vi "BeamProfiler.vi"() -> ()   [LabVIEW 2014]
uses:
  <vilib>/Analysis/6fits.llb/Curve Fitting Criteria.ctl
  <vilib>/vision/Image Controls.llb/IMAQ Rounding Mode.ctl
  <vilib>/vision/Image Controls.llb/IMAQ Image.ctl
  <vilib>/vision/NI_Vision_Development_Module.lvlib
  <vilib>/ptbypt/NI_PtbyPt.lvlib
  <vilib>/Analysis/NI_AALPro.lvlib
panel:
  in  "resample":dbl=1.0
  in  "Smooth":bool
  in  "max proj":bool
  in  "average":dbl=1.0
  in  "centroid":bool
  out "Temp":dbl format="%#_2g"
  out "fps":dbl
  in  "Exposure Time (ms)":dbl(slide)=32000.0 caption="Exposure Time" min=2000.0 max=32000.0 scale=2000.0..32000.0 scale format="%^#_3g"
  in  "Gain":dbl(slide)=1.0 min=1.0 max=4.0 scale=1.0..4.0
  in  "Auto":bool
  in  "Contrast":i64(slide) caption="Gain (Raw)" min=0 max=384 step=1 scale=0.0..100.0
  in  "Gamma":dbl(slide)=0.5 min=0.5 max=2.0 step=0.1 scale=0.5..2.0
  in  "Auto":bool
  out "Beam profile":T1(plugin-control)
  in  "zero":bool
  in  "mmPerPx":dbl=0.0059
  out "XY Center location":cluster{"Array":dbl[], "Array 3":dbl[]}(graph)
  out "Y center (px)":dbl
  out "X center (px)":dbl
  in  "Center\n Color":u32(colorbox)=10735
  in  "Black\n zero":bool=TRUE
  in  "Operator":T2(ring)=enum."Clear  if < "
  out "X Histogram":cluster{"X":dbl, "Y":dbl}[](graph)
  out "Y Histogram":cluster{"X":dbl, "Y":dbl}[](graph)
  in  "Palette Number (gray)":T3(ring)=enum."Rainbow"
  in  "Decrease":bool
  in  "Increase":bool
  in  "zoom 4":bool
  in  "zoom 3":bool
  in  "zoom 2":bool
  in  "zoom1":bool
  in  "stop":bool
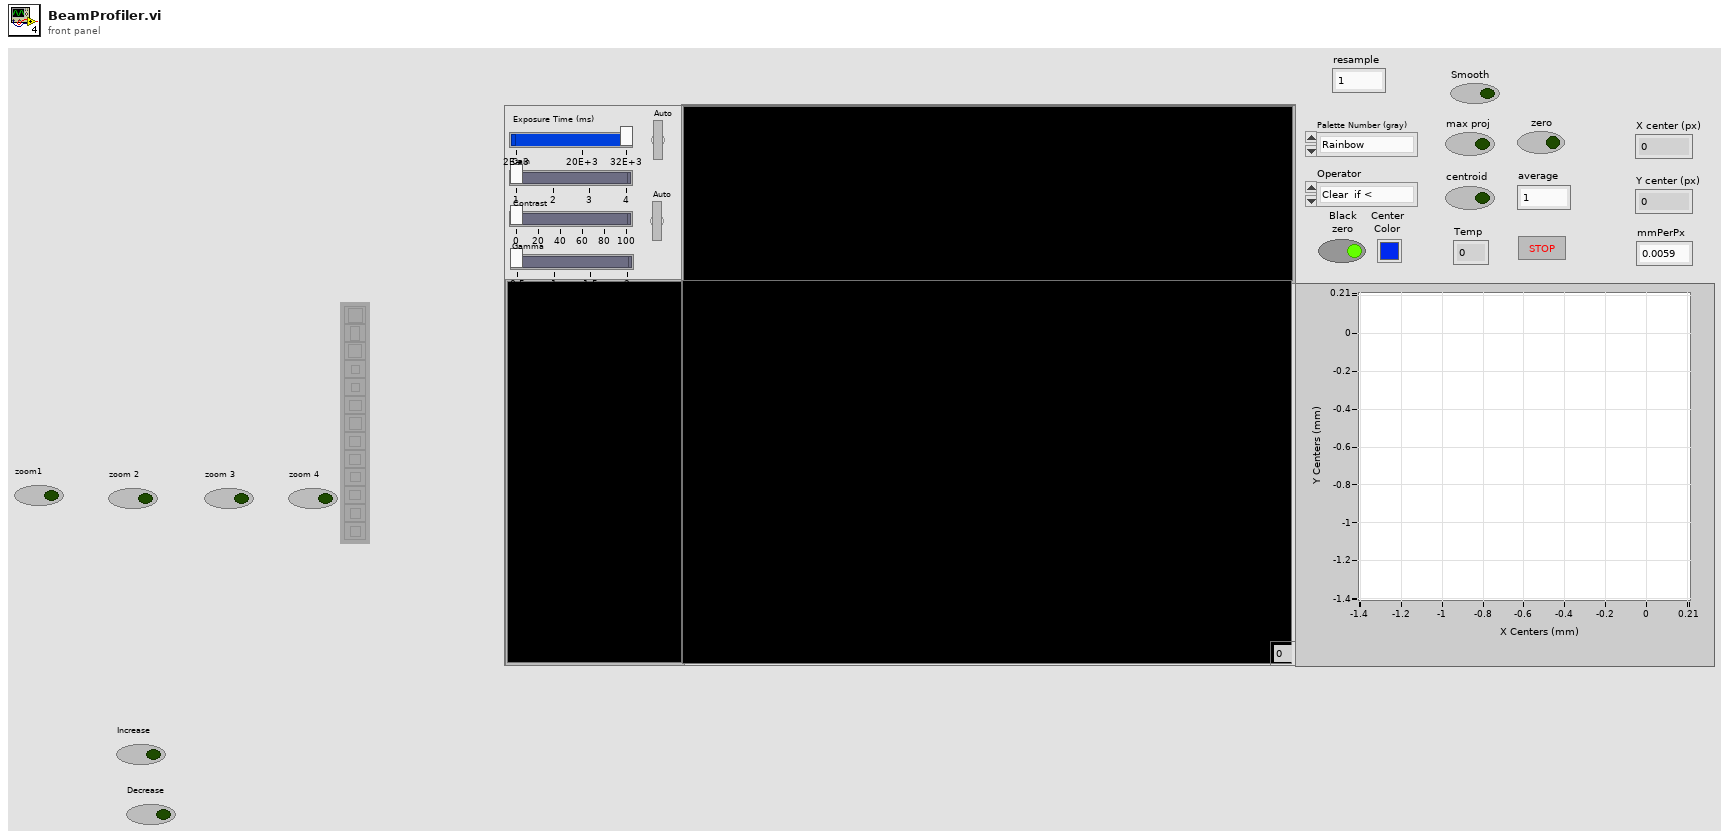
[diagram p1: front panel]
types:
  T1 = typedef "IMAQ Image.ctl" = refnum<image>
  T2 = enum32{"Average", "Min", "Max", "Clear  if < ", "Clear  if < or =", "Clear  if =", "Clear  if > or =", "Clear  if >"}
  T3 = enum32{"Gray", "Binary", "Gradient", "Rainbow", "Temperature"}
  T4 = typedef "Image Type" = u32
  T5 = typedef "IMAQ Rounding Mode.ctl" = enum16{"Optimize", "Truncate"}
  T6 = cluster{"Brightness":sgl, "Contrast":sgl, "Gamma":sgl}
  T7 = typedef "NI_AALPro.lvlib/Curve Fitting Criteria.ctl" = u16
  T8 = typedef "LVRangeTypeDef.ctl" = cluster{"Minimum":dbl, "Maximum":dbl, "Increment":dbl, "Minor Increment":dbl, "Start":dbl}
  T9 = cluster{"Mean Value":sgl, "Standard Variation":sgl, "Minimal Value":sgl, "Maximal Value":sgl, "Area (calibrated)":sgl, "Area (pixels)":u32, "%":sgl, "Calibration Valid":bool}
  T10 = typedef "ROI Descriptor" = cluster{"Global Rectangle":i32[], "Contours":cluster{"ID":enum32{"External", "Internal"}, "Type":u32, "Coordinates":i32[]}[]}
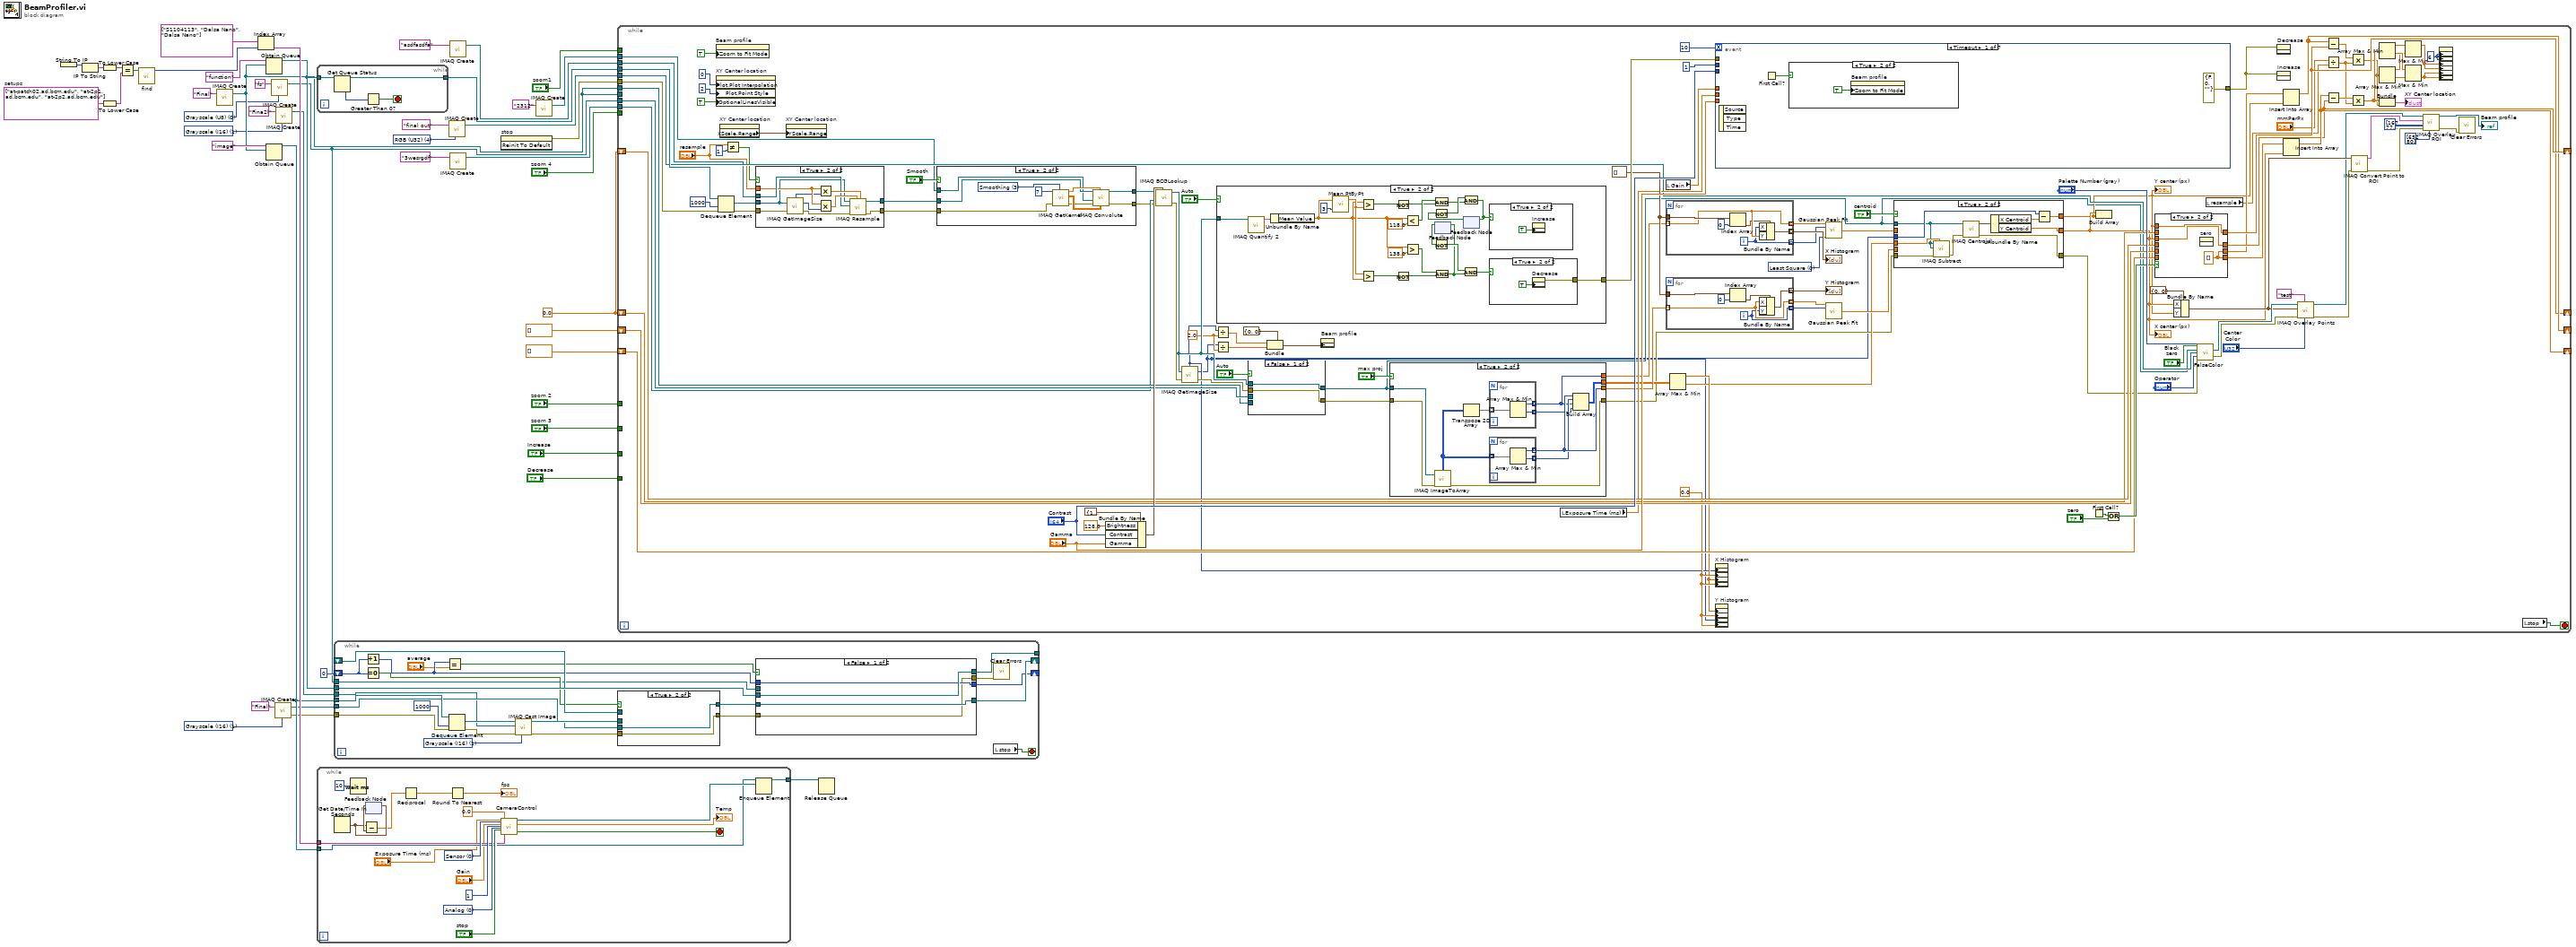
[diagram p0: block diagram]
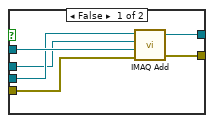
[diagram p2: hidden frame]
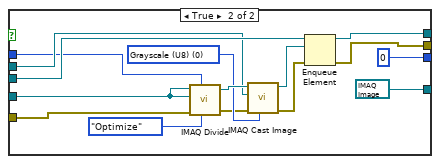
[diagram p3: hidden frame]
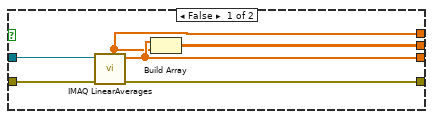
[diagram p6: hidden frame]
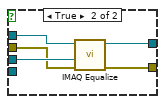
[diagram p9: hidden frame]
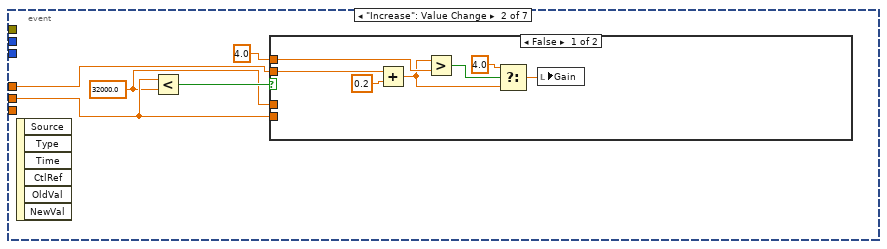
[diagram p14: hidden frame]
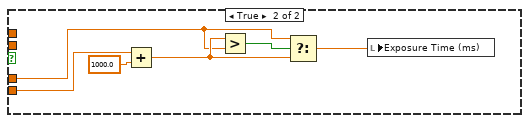
[diagram p15: hidden frame]
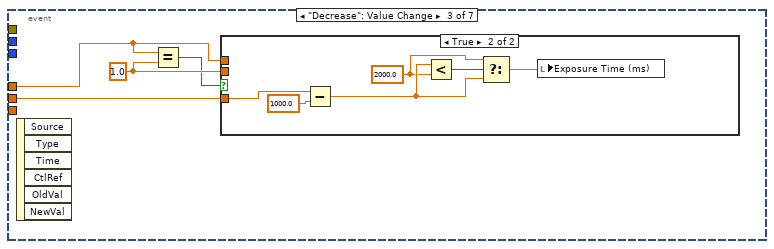
[diagram p16: hidden frame]
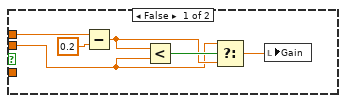
[diagram p17: hidden frame]
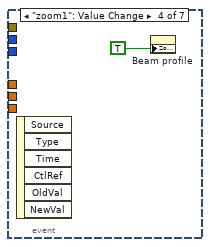
[diagram p18: hidden frame]
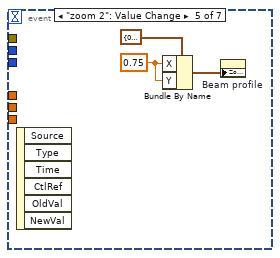
[diagram p19: hidden frame]
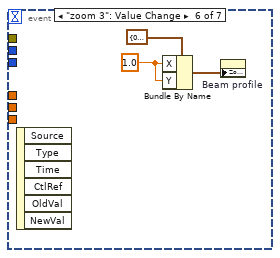
[diagram p20: hidden frame]
diagram:
  w9 = T4 0 items=["Grayscale (U8)", "Grayscale (I16)", "Grayscale (SGL)", "Complex (CSG)", "RGB (U32)", "HSL (U32)", "RGB (U64)", "Grayscale (U16)"] ("Image Type")
  w14 = T4 1 items=["Grayscale (U8)", "Grayscale (I16)", "Grayscale (SGL)", "Complex (CSG)", "RGB (U32)", "HSL (U32)", "RGB (U64)", "Grayscale (U16)"] ("Image Type")
  w16 = T4 1 items=["Grayscale (U8)", "Grayscale (I16)", "Grayscale (SGL)", "Complex (CSG)", "RGB (U32)", "HSL (U32)", "RGB (U64)", "Grayscale (U16)"] ("Image Type")
  w25 = T4 4 items=["Grayscale (U8)", "Grayscale (I16)", "Grayscale (SGL)", "Complex (CSG)", "RGB (U32)", "HSL (U32)", "RGB (U64)", "Grayscale (U16)"] ("Image Type")
  w29 = 0.0
  w36 = string[] ["at-patch02.ad.bcm.edu", "at-2p1.ad.bcm.edu", "at-2p2.ad.bcm.edu"]  # setups
  n1 = String To IP() -> (0:w39:u32)  [unwired: 1 in]
  n2 = IP To String(2:w39) -> (0:w38:string)  [unwired: 1 in]
  n3 = To Lower Case(string=w38) -> (all lower case string=w37:string)
  n4 = To Lower Case(string=w36) -> (all lower case string=w35:string[])
  n5 = Equal?(x=w37, y=w35) -> (x = y?=w34:bool[])
  n6 = call "find.vi"("Array"=w34) -> ("Index"=w33:i32)  [unwired: 10 in]
  n7 = call "IMAQ Create"("Image Name"="Final") -> ("New Image"=w18:T1)  [unwired: 4 in, 1 out]
  n8 = Index Array(array=string[] ["S1104113", "Dalsa Nano", "Dalsa Nano"], index=w33) -> (element=w28:string)
  n9 = Obtain Queue(name (unnamed)="function", element data type=w18) -> (queue out=w19:refnum<queue>)  [unwired: 3 in, 2 out]
  n10 = Obtain Queue(name (unnamed)="image", element data type=w18) -> (queue out=w20:refnum<queue>)  [unwired: 3 in, 2 out]
  n11 = call "IMAQ Create"("Image Name"="fs", "Image Type"=w9) -> ("New Image"=w8:T1)  [unwired: 3 in, 1 out]
  n12 = call "IMAQ Create"("Image Name"="Final", "Image Type"=w16) -> ("New Image"=w15:T1, "error out"=w7:errorcluster)  [unwired: 3 in]
  n13 = call "IMAQ Create"("Image Name"="Fina2l", "Image Type"=w14) -> ("New Image"=w12:T1)  [unwired: 3 in, 1 out]
  n14 = while {
    tunnel: w19 -> [w51]
    tunnel: [w50] -> w22
    stop <- w49 stop-if-true
    n15 = Get Queue Status(queue=w51) -> (queue out=w50:refnum<queue>, # elements in queue=w48:i32)  [unwired: 2 in, 6 out]
    n16 = Greater Than 0?(x=w48) -> (x > 0?=w49:bool)
  }
  n17 = while {
    tunnel: w28 -> [w65]
    tunnel: w20 -> [w62]
    tunnel: [w61] -> w27
    stop <- w64 stop-if-true
    w67 = u32 0 items=["Analog"] ("Black Level Selector")
    w66 = u32 0 items=["Sensor", "Digital"] ("Gain Selector")
    n18 = Get Date/Time In Seconds() -> (seconds since 1Jan1904=w56:timestamp)
    n19 = Wait (ms)(milliseconds to wait=u32 10) -> ()  [unwired: 1 out]
    n20 = feedback #1() -> (w57:timestamp)  [unwired: 1 in]
    n21 = Subtract(x=w56, y=w57) -> (x-y=w55:dbl)
    n22 = feedback-in #1(w56) -> ()
    n23 = Reciprocal(x=w55) -> (1/x=w58:dbl)
    n24 = Round To Nearest(number=w58) -> (nearest integer value=→"fps":dbl)
    n25 = call "CameraControl.vi"("Exposure Time"="Exposure Time (ms)", "Gain Selector"=w66, "Gain"="Gain", "Gain (Raw)"=i64 1, "Black Level Selector"=w67, "Stop (F)"="stop", "Black Level"=0.0, "Camera"=w65) -> ("Image Out"=w63:T1, "Temp"=→"Temp":dbl, "Stopped"=w64:bool)  [unwired: 14 in, 3 out]
    n26 = Enqueue Element(queue=w62, element=w63) -> (queue out=w61:refnum<queue>)  [unwired: 2 in, 2 out]
  }
  n27 = while {
    tunnel: w19 -> [w93]
    tunnel: w20 -> [w94]
    tunnel: [w92] -> _
    shift-right: [w84] -> _
    shift-left: _ -> [w91]
    tunnel: w15 -> [w90]
    tunnel: w12 -> [w87]
    shift-right: [w83] -> _
    shift-left: 0 -> [w79]
    tunnel: w8 -> [w77]
    tunnel: w7 -> [w75]
    stop <- w95 stop-if-true
    w86 = T4 1 items=["Grayscale (U8)", "Grayscale (I16)", "Grayscale (SGL)", "Complex (CSG)", "RGB (U32)", "HSL (U32)", "RGB (U64)", "Grayscale (U16)"] ("Image Type")
    n28 = Increment(x=w79) -> (x+1=w80:i32)
    n29 = Equal To 0?(x=w79) -> (x = 0?=w82:bool)
    n30 = Equal?(x=w80, y="average") -> (x = y?=w81:bool)
    n31 = Dequeue Element(queue=w94, timeout in ms (-1)=1000, error in (no error)=w75) -> (element=w88:T1, error out=w74:errorcluster)  [unwired: 2 out]
    n32 = call "IMAQ Cast Image"("Image Type"=w86, "error in (no error)"=w74, "Image Dst"=w87, "Image Src"=w88) -> ("error out"=w73:errorcluster, "Image Dst Out"=w89:T1)  [unwired: 6 in]
    n33 = case shown="True" w82 {
      tunnel: w89 -> [w100 w103]
      tunnel: [w99 w103] -> w85
      tunnel: w91 -> [w101 _]
      tunnel: w90 -> [w98 _]
      tunnel: w73 -> [w97 w102]
      tunnel: [w96 w102] -> w72
      frame False {
        n34 = call "IMAQ Add"("Image Src A"=w100, "Image Dst"=w98, "Image Src B"=w101, "error in (no error)"=w97) -> ("Image Dst Out"=w99:T1, "error out"=w96:errorcluster)  [unwired: 3 in]
      }
      frame True {
      }
    }
    n35 = case shown="False" w81 {
      tunnel: w93 -> [w107 w122]
      tunnel: [w107 w121] -> w92
      tunnel: w85 -> [w106 w112]
      tunnel: [w106 T1 refnum ("Image Dst Out")] -> w84
      tunnel: w80 -> [w105 w113]
      tunnel: [w105 0] -> w83
      tunnel: w77 -> [_ w114]
      tunnel: w72 -> [w104 w111]
      tunnel: [w104 w108] -> w71
      frame False {
      }
      frame True {
        w115 = T4 0 items=["Grayscale (U8)", "Grayscale (I16)", "Grayscale (SGL)", "Complex (CSG)", "RGB (U32)", "HSL (U32)", "RGB (U64)", "Grayscale (U16)"] ("Image Type")
        n36 = call "IMAQ Divide"("Image Src A"=w112, "Constant"=w113, "Image Dst"=w112, "Rounding Mode"=IMAQ_Rounding_Mode."Optimize", "error in (no error)"=w111) -> ("Image Dst Out"=w116:T1, "error out"=w110:errorcluster)  [unwired: 2 in]
        n37 = call "IMAQ Cast Image"("Image Type"=w115, "error in (no error)"=w110, "Image Dst"=w114, "Image Src"=w116) -> ("error out"=w109:errorcluster, "Image Dst Out"=w117:T1)  [unwired: 6 in]
        n38 = Enqueue Element(queue=w122, element=w117, error in (no error)=w109) -> (queue out=w121:refnum<queue>, error out=w108:errorcluster)  [unwired: 1 in, 1 out]
      }
    }
    n39 = call <vilib>:"Clear Errors.vi"("error in (no error)"=w71) -> ()  [unwired: 5 in, 2 out]
    n40 = local read "stop"() -> (w95:bool)
  }
  n41 = call "IMAQ Create"("Image Name"="final out", "Image Type"=w25) -> ("New Image"=w23:T1)  [unwired: 3 in, 1 out]
  n42 = call "IMAQ Create"("Image Name"="asdfasdfa") -> ("New Image"=w1:T1)  [unwired: 4 in, 1 out]
  n43 = call "IMAQ Create"("Image Name"="3wesrgdf") -> ("New Image"=w5:T1)  [unwired: 4 in, 1 out]
  n44 = invoke on="stop" class="Bool (strict)" method="Reinit To Default"() -> (error out=w40:errorcluster)  [unwired: 3 in, 2 out]
  n45 = call "IMAQ Create"("Image Name"="2312") -> ("New Image"=w3:T1)  [unwired: 4 in, 1 out]
  n46 = while {
    tunnel: "zoom1" -> [_]
    tunnel: "zoom 4" -> [_]
    tunnel: "zoom 2" -> [_]
    tunnel: "zoom 3" -> [_]
    tunnel: "Increase" -> [_]
    tunnel: "Decrease" -> [_]
    tunnel: w18 -> [w146]
    tunnel: w40 -> [w149]
    shift-right: [w201] -> _
    shift-left: dbl[] [] -> [w190]
    shift-right: [w199] -> _
    shift-left: dbl[] [] -> [w192]
    shift-right: [w198] -> _
    shift-left: w29 -> [w202]
    shift-right: [w200] -> _
    shift-left: w29 -> [w203]
    tunnel: w22 -> [w175]
    tunnel: w23 -> [w174]
    tunnel: w18 -> [_]
    tunnel: w8 -> [w164]
    tunnel: w5 -> [w145]
    tunnel: w3 -> [w141]
    tunnel: w1 -> [w136]
    stop <- w176 stop-if-true
    w127 = 2.0 ("y")
    w172 = 0.0 ("X Scale.Range:Minimum")
    w188 = u8 6 ("X Scale.Mapping Mode")
    w193 = T7 0 items=["Least Square", "Least Absolute Residual", "Bisquare"] ("method")
    w226 = cluster{"X":dbl, "Y":dbl}[] [] ("XY Graph")
    n47 = property on="Beam profile" class="ImageControl"("Zoom to Fit Mode"=TRUE) -> ()  [unwired: 2 in, 2 out]
    n48 = property on="XY Center location" class="XYGraph (strict)"("Plot.Plot Interpolation"=u8 0, "Plot.Point Style"=u8 2 ("Cursor.Cursor Point Style"), "OptionalLinesVisible"=TRUE ("Cartesian Lines:Visible")) -> ()  [unwired: 2 in, 2 out]
    n49 = Dequeue Element(queue=w175, timeout in ms (-1)=1000, error in (no error)=w149) -> (element=w138:T1, error out=w131:errorcluster)  [unwired: 2 out]
    n50 = property on="XY Center location" class="XYGraph (strict)"() -> ("XScale.Range"=w173:T8)  [unwired: 2 in, 2 out]
    n51 = Not Equal?(x="resample", y=1) -> (x != y?=w133:bool)
    n52 = case shown="True" w133 {
      tunnel: w138 -> [w241 w244]
      tunnel: [w241 w252] -> w140
      tunnel: w131 -> [w240 w243]
      tunnel: [w240 w251] -> w139
      tunnel: w136 -> [_ w248]
      tunnel: "resample" -> [_ w247]
      frame False {
      }
      frame True {
        n53 = call "IMAQ GetImageSize"("Image"=w244, "error in (no error)"=w243) -> ("Y Resolution"=w245:i32, "X Resolution"=w246:i32, "error out"=w242:errorcluster)  [unwired: 2 in]
        n54 = Multiply(x=w247, y=w246) -> (x*y=w249:dbl)
        n55 = Multiply(x=w247, y=w245) -> (x*y=w250:dbl)
        n56 = call "IMAQ Resample"("X Resolution"=w249, "Y Resolution"=w250, "error in (no error)"=w242, "Image Dst"=w248, "Image Src"=w244) -> ("error out"=w251:errorcluster, "Image Dst Out"=w252:T1)  [unwired: 5 in]
      }
    }
    n57 = property on="XY Center location" class="XYGraph (strict)"("YScale.Range"=w173) -> ()  [unwired: 2 in, 2 out]
    n58 = case shown="True" "Smooth" {
      tunnel: [w254 w261] -> w144
      tunnel: w139 -> [w254 w260]
      tunnel: [w253 w258] -> w143
      tunnel: w140 -> [w253 w259]
      tunnel: w141 -> [_ w256]
      frame False {
      }
      frame True {
        w255 = u16 3 items=["Gradient"=1, "Laplacian"=2, "Smoothing"=3, "Gaussian"=4] ("Kernel Family")
        n59 = call "IMAQ GetKernel"("Kernel Family"=w255, "error in (no error)"=w260, "Kernel Size (3,5,...)"=7) -> ("error out"=w262:errorcluster, "Kernel"=w264:sgl[][], "Divider"=w263:sgl)  [unwired: 5 in, 1 out]
        n60 = call "IMAQ Convolute"("Kernel"=w264, "Divider (kernel sum)"=w263, "error in (no error)"=w262, "Image Dst"=w256, "Image Src"=w259) -> ("error out"=w261:errorcluster, "Image Dst Out"=w258:T1)  [unwired: 5 in]
      }
    }
    n61 = Bundle By Name(cluster=T6 {"Brightness"=128.0, "Contrast"=45.0, "Gamma"=1.0} ("BCG Values"), "Brightness"=sgl 128.0, "Contrast"="Contrast", "Gamma"="Gamma") -> (w230:T6)
    n62 = call "IMAQ BCGLookup"("Image Src"=w143, "BCG Values"=w230, "Image Dst"=w145, "error in (no error)"=w144) -> ("Image Dst Out"=w147:T1, "error out"=w148:errorcluster)  [unwired: 3 in]
    n63 = call "IMAQ GetImageSize"("Image"=w147, "error in (no error)"=w148) -> ("Y Resolution"=w123:i32, "X Resolution"=w124:i32, "error out"=w157:errorcluster)  [unwired: 2 in]
    n64 = Divide(x=w124, y=w127) -> (x/y=w126:dbl)
    n65 = Divide(x=w123, y=w127) -> (x/y=w125:dbl)
    n66 = case shown="True" "Auto" {
      tunnel: w147 -> [_ w347]
      tunnel: [_ w345] -> w237
      frame False {
      }
      frame True {
        n67 = call "IMAQ Quantify 2"("Image"=w347) -> ("Global Report"=w343:T9)  [unwired: 8 in, 2 out]
        n68 = Unbundle By Name(w343) -> ("Mean Value"=w335:sgl)
        n69 = call <vilib>:"Mean PtByPt.vi"("x"=w335, "sample length"=3) -> ("mean"=w336:dbl)  [unwired: 2 in, 1 out]
        n70 = Greater?(x=w335, y=w336) -> (0:w340:bool)
        n71 = Greater?(x=w336, y=w335) -> (0:w337:bool)
        n72 = Not(x=w340) -> (.not. x?=w339:bool)
        n73 = Not(x=w337) -> (.not. x?=w338:bool)
        n74 = Less?(x=w335, y=sgl 118.0) -> (x < y?=w342:bool)
        n75 = Greater?(x=w335, y=sgl 138.0) -> (0:w328:bool)
        n76 = And(x=w342, y=w339) -> (x .and. y?=w332:bool)
        n77 = feedback #2() -> (w329:bool)  [unwired: 1 in]
        n78 = Not(x=w329) -> (.not. x?=w330:bool)
        n79 = And(x=w328, y=w338) -> (x .and. y?=w327:bool)
        n80 = feedback-in #2(w327) -> ()
        n81 = And(x=w330, y=w327) -> (x .and. y?=w326:bool)
        n82 = feedback #3() -> (w334:bool)  [unwired: 1 in]
        n83 = Not(x=w334) -> (.not. x?=w333:bool)
        n84 = And(x=w333, y=w332) -> (x .and. y?=w331:bool)
        n85 = feedback-in #3(w331) -> ()
        n86 = case shown="True" w331 {
          frame False {
          }
          frame True {
            n87 = property on="Increase" class="Bool (strict)"("Val(Sgnl)"=TRUE ("Value (Signaling)")) -> ()  [unwired: 2 in, 2 out]
          }
        }
        n88 = case shown="True" w326 {
          tunnel: [_ w349] -> w345
          frame False {
          }
          frame True {
            n89 = property on="Decrease" class="Bool (strict)"("Val(Sgnl)"=TRUE ("Value (Signaling)")) -> (error out=w349:errorcluster)  [unwired: 2 in, 1 out]
          }
        }
      }
    }
    n90 = case shown="False" "Auto" {
      tunnel: [w320 w324] -> w159
      tunnel: w147 -> [w320 w325]
      tunnel: w146 -> [_ _]
      tunnel: w164 -> [_ w323]
      tunnel: w157 -> [w319 w322]
      tunnel: [w319 w321] -> w156
      frame False {
      }
      frame True {
        n91 = call "IMAQ Equalize"("error in (no error)"=w322, "Image Dst"=w323, "Image Src"=w325) -> ("error out"=w321:errorcluster, "Image Dst Out"=w324:T1)  [unwired: 7 in]
      }
    }
    n92 = Bundle(cluster=cluster{"X":u32, "Y":u32} {"X"=0, "Y"=0} ("Image Center Position:All Elements"), "X"=w126, "Y"=w125) -> (w128:cluster{"X":u32, "Y":u32})
    n93 = property on="Beam profile" class="ImageControl"("Image Center Position"=w128) -> ()  [unwired: 2 in, 2 out]
    n94 = case shown="True" "max proj" {
      tunnel: [w268 w275] -> w162
      tunnel: [w269 w277] -> w161
      tunnel: w159 -> [w270 w280]
      tunnel: [w267 w273] -> w158
      tunnel: w156 -> [w266 w272]
      tunnel: [w265 w271] -> w155
      frame False {
        n95 = call "IMAQ LinearAverages"("error in (no error)"=w266, "Image Src"=w270) -> ("error out"=w265:errorcluster, "Y Axis Averages"=w269:sgl[], "X Axis Averages"=w268:sgl[])  [unwired: 5 in, 2 out]
        n96 = Build Array(w269, w268) -> (w267:sgl[][])
      }
      frame True {
        n97 = call "IMAQ ImageToArray"("error in (no error)"=w272, "Image"=w280) -> ("error out"=w271:errorcluster, "Image Pixels (U8)"=w279:u8[][])  [unwired: 2 in, 3 out]
        n98 = Transpose 2D Array(2D array=w279) -> (transposed array=w278:u8[][])
        n99 = for {
          tunnel: w278 -> [w283] mode=indexing
          tunnel: [w282] -> w275 mode=indexing
          tunnel: [w281] -> w274 mode=indexing
          n100 = Array Max & Min(array=w283) -> (max value=w282:u8, min value=w281:u8)  [unwired: 2 out]
        }
        n101 = for {
          tunnel: w279 -> [w286] mode=indexing
          tunnel: [w285] -> w277 mode=indexing
          tunnel: [w284] -> w276 mode=indexing
          n102 = Array Max & Min(array=w286) -> (max value=w285:u8, min value=w284:u8)  [unwired: 2 out]
        }
        n103 = Build Array(w277, w276, w275, w274) -> (w273:u8[][])
      }
    }
    n104 = local read "Exposure Time (ms)"() -> (w179:dbl)
    n105 = local read "Gain"() -> (w178:dbl)
    n106 = for {
      tunnel: w226 -> [w312]
      tunnel: w162 -> [w309] mode=indexing
      tunnel: [w310] -> w227 mode=indexing
      tunnel: [w309] -> w214 mode=indexing
      tunnel: [w308] -> w213 mode=indexing
      i -> [w308]
      n107 = Index Array(array=w312, index=0) -> (element=w307:cluster{"X":dbl, "Y":dbl})
      n108 = Bundle By Name(cluster=w307, "X"=w308, "Y"=w309) -> (w310:cluster{"X":dbl, "Y":dbl})
    }
    "X Histogram" <- w227
    n109 = for {
      tunnel: w226 -> [w318]
      tunnel: w161 -> [w314] mode=indexing
      tunnel: [w315] -> w228 mode=indexing
      tunnel: [w314] -> w212 mode=indexing
      tunnel: [w313] -> w211 mode=indexing
      i -> [w313]
      n110 = Index Array(array=w318, index=0) -> (element=w316:cluster{"X":dbl, "Y":dbl})
      n111 = Bundle By Name(cluster=w316, "X"=w314, "Y"=w313) -> (w315:cluster{"X":dbl, "Y":dbl})
    }
    "Y Histogram" <- w228
    n112 = Array Max & Min(array=w158) -> (max value=w166:sgl, min value=w163:sgl)  [unwired: 2 out]
    n113 = event shown="[0] Timeout" {
      selector: _ -> [_ _ _ _ _ _ _]
      dyn-events: _ -> [_ _ _ _ _ _ _]
      timeout: 10 -> [_ _ _ _ _ _ _]
      tunnel: w179 -> [_ w356 w373 _ _ _ _]
      tunnel: i64 1 ("Gain (Raw)") -> [_ _ _ _ _ _ _]
      tunnel: w178 -> [_ w358 w374 _ _ _ _]
      tunnel: "Contrast" -> [_ _ _ _ _ _ _]
      tunnel: "Gamma" -> [_ _ _ _ _ _ _]
      tunnel: [errorcluster {"status"=FALSE, "code"=0, "source"=""} ("error out") _ _ _ _ _ _] -> w238
      tunnel: w237 -> [_ _ _ _ _ _ _]
      event Timeout {
        n114 = event-data() -> ()  [unwired: 1 in, 3 out]
        n115 = First Call?() -> (First Call?: T/F=w351:bool)
        n116 = case shown="True" w351 {
          frame False {
          }
          frame True {
            n117 = property on="Beam profile" class="ImageControl"("Zoom to Fit Mode"=TRUE) -> ()  [unwired: 2 in, 2 out]
          }
        }
      }
      event "Increase": Value Change {
        w354 = 32000.0 ("y")
        n118 = event-data() -> ()  [unwired: 1 in, 6 out]
        n119 = Less?(x=w356, y=w354) -> (x < y?=w355:bool)
        n120 = case shown="False" w355 {
          tunnel: w356 -> [_ w371]
          tunnel: w358 -> [w365 _]
          tunnel: 4.0 ("y") -> [w363 _]
          tunnel: w354 -> [_ w366]
          frame False {
            n121 = Add(x=w365, y=0.2) -> (x+y=w361:dbl)
            n122 = Greater?(x=w361, y=w363) -> (0:w362:bool)
            n123 = Select(t=4.0, s=w362, f=w361) -> (s? t:f=w359:dbl)
            n124 = local write "Gain"(w359) -> ()
          }
          frame True {
            n125 = Add(x=w371, y=1000.0) -> (x+y=w368:dbl)
            n126 = Greater?(x=w368, y=w366) -> (0:w369:bool)
            n127 = Select(t=w366, s=w369, f=w368) -> (s? t:f=w367:dbl)
            n128 = local write "Exposure Time (ms)"(w367) -> ()
          }
        }
      }
      event "Decrease": Value Change {
        w375 = 1.0 ("y")
        n129 = event-data() -> ()  [unwired: 1 in, 6 out]
        n130 = Equal?(x=w374, y=w375) -> (x = y?=w372:bool)
        n131 = case shown="True" w372 {
          tunnel: w373 -> [_ w387]
          tunnel: w374 -> [w381 _]
          tunnel: w375 -> [w376 _]
          frame False {
            n132 = Subtract(x=w381, y=0.2) -> (x-y=w378:dbl)
            n133 = Less?(x=w378, y=w376) -> (x < y?=w379:bool)
            n134 = Select(t=w376, s=w379, f=w378) -> (s? t:f=w377:dbl)
            n135 = local write "Gain"(w377) -> ()
          }
          frame True {
            w383 = 2000.0 ("y")
            n136 = Subtract(x=w387, y=1000.0) -> (x-y=w384:dbl)
            n137 = Less?(x=w384, y=w383) -> (x < y?=w385:bool)
            n138 = Select(t=w383, s=w385, f=w384) -> (s? t:f=w382:dbl)
            n139 = local write "Exposure Time (ms)"(w382) -> ()
          }
        }
      }
      event "zoom1": Value Change {
        n140 = event-data() -> ()  [unwired: 1 in, 6 out]
        n141 = property on="Beam profile" class="ImageControl"("Zoom to Fit Mode"=TRUE) -> ()  [unwired: 2 in, 2 out]
      }
      event "zoom 2": Value Change {
        w389 = 0.75
        n142 = event-data() -> ()  [unwired: 1 in, 6 out]
        n143 = Bundle By Name(cluster=cluster{"X":sgl, "Y":sgl} {"X"=0.0, "Y"=0.0} ("ZoomSingle:All Elements"), "X"=w389, "Y"=w389) -> (w391:cluster{"X":sgl, "Y":sgl})
        n144 = property on="Beam profile" class="ImageControl"("ZoomSingle"=w391) -> ()  [unwired: 2 in, 2 out]
      }
      event "zoom 3": Value Change {
        w392 = 1.0
        n145 = event-data() -> ()  [unwired: 1 in, 6 out]
        n146 = Bundle By Name(cluster=cluster{"X":sgl, "Y":sgl} {"X"=0.0, "Y"=0.0} ("ZoomSingle:All Elements"), "X"=w392, "Y"=w392) -> (w394:cluster{"X":sgl, "Y":sgl})
        n147 = property on="Beam profile" class="ImageControl"("ZoomSingle"=w394) -> ()  [unwired: 2 in, 2 out]
      }
      event "zoom 4": Value Change {
        w395 = 1.5
        n148 = event-data() -> ()  [unwired: 1 in, 6 out]
        n149 = Bundle By Name(cluster=cluster{"X":sgl, "Y":sgl} {"X"=0.0, "Y"=0.0} ("ZoomSingle:All Elements"), "X"=w395, "Y"=w395) -> (w397:cluster{"X":sgl, "Y":sgl})
        n150 = property on="Beam profile" class="ImageControl"("ZoomSingle"=w397) -> ()  [unwired: 2 in, 2 out]
      }
    }
    n151 = property on="X Histogram" class="XYGraph (strict)"("XScale.Maximum"=w124, "XScale.Minimum"=w172, "YScale.Maximum"=w166, "YScale.Minimum"=w172) -> ()  [unwired: 2 in, 2 out]
    n152 = property on="Y Histogram" class="XYGraph (strict)"("XScale.Maximum"=w166, "XScale.Minimum"=w172, "YScale.Maximum"=w123, "YScale.Minimum"=w172) -> ()  [unwired: 2 in, 2 out]
    n153 = call <vilib>:"Gaussian Peak Fit.vi"("Y"=w214, "X"=w213, "method"=w193) -> ("center"=w170:dbl)  [unwired: 6 in, 6 out]
    n154 = call <vilib>:"Gaussian Peak Fit.vi"("Y"=w212, "X"=w211) -> ("center"=w168:dbl)  [unwired: 7 in, 6 out]
    n155 = case shown="True" "centroid" {
      tunnel: w170 -> [w289 _]
      tunnel: [w289 w295] -> w169
      tunnel: w168 -> [w288 _]
      tunnel: [w288 w298] -> w167
      tunnel: w123 -> [_ w299]
      tunnel: w159 -> [_ w290]
      tunnel: w163 -> [_ w294]
      tunnel: w155 -> [w287 w293]
      tunnel: [w287 w291] -> w153
      frame False {
      }
      frame True {
        n156 = call "IMAQ Subtract"("Image Src A"=w290, "Constant"=w294, "Image Dst"=w290, "error in (no error)"=w293) -> ("error out"=w292:errorcluster)  [unwired: 3 in, 1 out]
        n157 = call "IMAQ Centroid"("error in (no error)"=w292, "Image"=w290) -> ("error out"=w291:errorcluster, "Centroid"=w297:cluster{"X Centroid":sgl, "Y Centroid":sgl})  [unwired: 2 in]
        n158 = Unbundle By Name(w297) -> ("X Centroid"=w296:sgl, "Y Centroid"=w295:sgl)
        n159 = Subtract(x=w299, y=w296) -> (x-y=w298:sgl)
      }
    }
    "X center (px)" <- w169
    "Y center (px)" <- w167
    n160 = First Call?() -> (First Call?: T/F=w205:bool)
    n161 = Build Array(w169, w167) -> ()  [unwired: 1 out]
    n162 = Or(x=w205, y="zero") -> (x .or. y?=w206:bool)
    n163 = case shown="True" w206 {
      tunnel: w203 -> [w303 _]
      tunnel: [w303 w306] -> w200
      tunnel: [w302 w305] -> w198
      tunnel: w202 -> [w302 _]
      tunnel: w169 -> [_ w306]
      tunnel: w167 -> [_ w305]
      tunnel: w192 -> [w301 _]
      tunnel: [w301 w304] -> w191
      tunnel: w190 -> [w300 _]
      tunnel: [w300 w304] -> w189
      frame False {
      }
      frame True {
        w304 = dbl[] []
        n164 = invoke on="zero" class="Bool (strict)" method="Reinit To Default"() -> ()  [unwired: 3 in, 3 out]
      }
    }
    n165 = Bundle By Name(cluster=cluster{"X":i32, "Y":i32} {"X"=0, "Y"=0} ("Point"), "X"=w169, "Y"=w167) -> (w219:cluster{"X":i32, "Y":i32})
    n166 = call "FalseColor.vi"("Black zero"="Black\n zero", "Palette Number (gray)"="Palette Number (gray)", "Image"=w159, "Image Dst"=w174, "Operator"="Operator", "error in (no error)"=w153) -> ("Image Dst Out"=w223:T1, "error out"=w152:errorcluster)  [unwired: 8 in]
    n167 = local read "resample"() -> (w137:dbl)
    n168 = invoke on="Decrease" class="Bool (strict)" method="Reinit To Default"(error in=w238) -> ()  [unwired: 2 in, 3 out]
    n169 = invoke on="Increase" class="Bool (strict)" method="Reinit To Default"(error in=w238) -> ()  [unwired: 2 in, 3 out]
    n170 = Insert Into Array(array=w191, new element=w167) -> (w199:dbl[])  [unwired: 1 in]
    n171 = Insert Into Array(array=w189, new element=w169) -> (w201:dbl[])  [unwired: 1 in]
    n172 = call "IMAQ Overlay Points"("Color"="Center\n Color", "Group"="test", "error in (no error)"=w152, "Point"=w219, "Image"=w223) -> ("error out"=w154:errorcluster, "Image Out"=w218:T1)  [unwired: 5 in]
    n173 = Subtract(x=w199, y=w198) -> (x-y=w196:dbl[])
    n174 = Divide(x="mmPerPx", y=w137) -> (x/y=w194:dbl)
    n175 = Subtract(x=w201, y=w200) -> (x-y=w197:dbl[])
    n176 = Multiply(x=w196, y=w194) -> (x*y=w180:dbl[])
    n177 = Multiply(x=w197, y=w194) -> (x*y=w181:dbl[])
    n178 = call "IMAQ Convert Point to ROI"("error in (no error)"=w154, "Point"=w219) -> ("error out"=w151:errorcluster, "ROI Descriptor"=w217:T10)  [unwired: 7 in]
    n179 = Array Max & Min(array=w181) -> (max value=w182:dbl, min value=w185:dbl)  [unwired: 2 out]
    n180 = Array Max & Min(array=w180) -> (max value=w183:dbl, min value=w184:dbl)  [unwired: 2 out]
    n181 = Bundle(w181, w180) -> (→"XY Center location":cluster{dbl[], dbl[]})  [unwired: 1 in]
    n182 = Max & Min(x=w182, y=w183) -> (max(x,y)=w187:dbl)  [unwired: 1 out]
    n183 = Max & Min(x=w185, y=w184) -> (min(x,y)=w186:dbl)  [unwired: 1 out]
    n184 = call "IMAQ Overlay ROI"("Colors (Green)"=u32[] [65280], "error in (no error)"=w151, "Point Symbol"=u32[][] [[16777216, 16777216, 16777216, 0, 16777216, 16777216, 16777216], [16777216, 16777216, 16777216, 0, 16777216, 16777216, 16777216], [16777216, 16777216, 16777216, 0, 16777216, 16777216, 16777216], [0, 0, 0, 0, 0, 0, 0], [16777216, 16777216, 16777216, 0, 16777216, 16777216, 16777216], [16777216, 16777216, 16777216, 0, 16777216, 16777216, 16777216], [16777216, 16777216, 16777216, 0, 16777216, 16777216, 16777216]], "ROI Descriptor"=w217, "Image"=w218) -> ("error out"=w150:errorcluster, "Image Out"=→"Beam profile":T1)  [unwired: 5 in]
    n185 = property on="XY Center location" class="XYGraph (strict)"("XScale.Style"=w188, "YScale.Style"=w188, "XScale.Maximum"=w187, "YScale.Maximum"=w187, "YScale.Minimum"=w186, "XScale.Minimum"=w186) -> ()  [unwired: 2 in, 2 out]
    n186 = call <vilib>:"Clear Errors.vi"("error in (no error)"=w150) -> ()  [unwired: 5 in, 2 out]
    n187 = local read "stop"() -> (w176:bool)
  }
  n188 = Release Queue(queue=w27) -> ()  [unwired: 2 in, 3 out]
